vi "Actuators Messenger Template.vi"(0 "Notifier Name":string, 11 "Error In":errorcluster) -> (4 "Notifier Name Out":string, 15 "Error Out":errorcluster)   [LabVIEW 2020]
uses:
  Actuators Controls/Actuators Actions.ctl
  Actuators Controls/Actuators Note Type.ctl
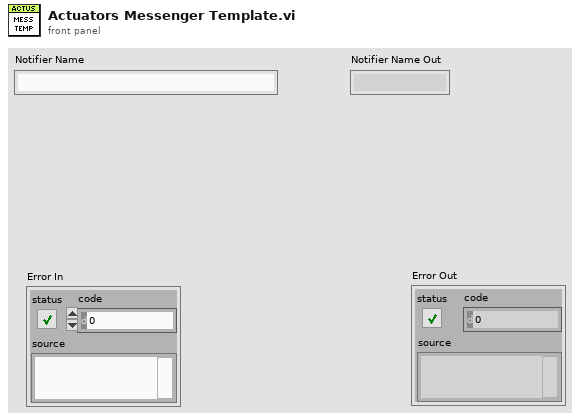
[diagram p1: front panel]
types:
  T1 = typedef "Actuators Note Type.ctl" = cluster{"Actions":T2, "Cmd Received ":bool, "Setpoint":dbl[], "Position":dbl[], "Channel":i32[], "Jog Step":dbl[], "Velocity":dbl[], "Acceleration":dbl[]}
  T2 = typedef "Actuators Actions.ctl" = enum16{"Nothing", "Get Position", "Get Acceleration", "Get Velocity", "Get Jog Step", "Set Acceleration", "Set Velocity", "Set Jog Step", "Move Absolute", "Move Relative", "Jog Forward", "Jog Reverse", "Halt", "Quit"}
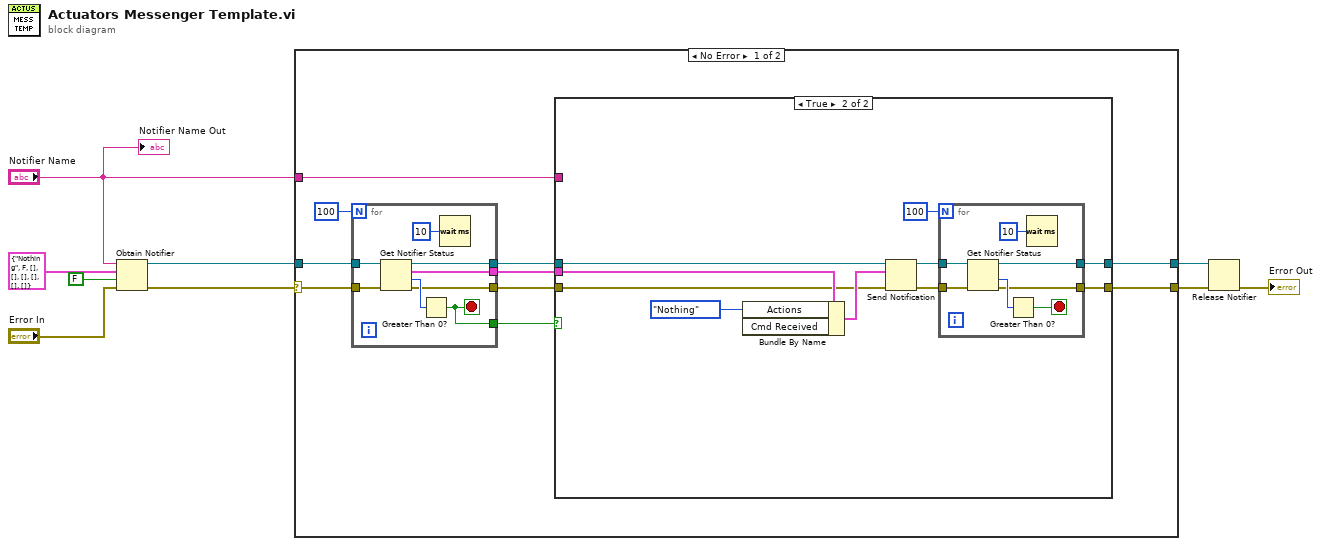
[diagram p0: block diagram]
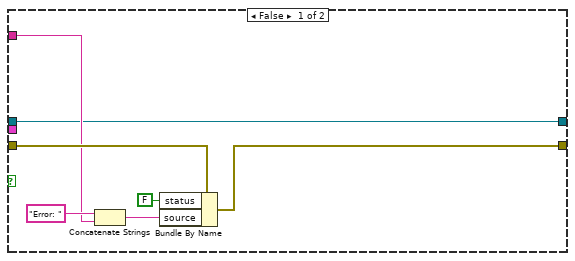
[diagram p2: hidden frame]
diagram:
  n1 = Obtain Notifier(name (unnamed)="Notifier Name", notification data type=T1 {"Actions"=enum."Nothing", "Cmd Received "=FALSE, "Setpoint"=[], "Position"=[], "Channel"=[], "Jog Step"=[], "Velocity"=[], "Acceleration"=[]} ("Actuators Note"), create if not found? (T)=FALSE, error in (no error)="Error In") -> (notifier out=w5:refnum<notifier>, error out=w8:errorcluster)  [unwired: 1 out]
  n2 = case shown="No Error" w8 {
    selector: w8 -> [w17 w52]
    tunnel: w5 -> [w18 w53]
    tunnel: "Notifier Name" -> [w12 _]
    tunnel: [w11 w53] -> w4
    tunnel: [w10 w52] -> w3
    frame No Error {
      n3 = for {
        N: 100 -> [_]
        tunnel: [w50] -> w14
        tunnel: w18 -> [w51]
        tunnel: [w49] -> w15
        tunnel: w17 -> [w46]
        tunnel: [w45] -> w16
        tunnel: [w44] -> w13
        stop <- w45 stop-if-true
        n4 = Get Notifier Status(notifier=w51, error in (no error)=w46) -> (notifier out=w49:refnum<notifier>, current notification=w50:T1, # waiting=w48:i32, error out=w44:errorcluster)  [unwired: 1 out]
        n5 = Greater Than 0?(x=w48) -> (x > 0?=w45:bool)
        n6 = Wait (ms)(milliseconds to wait=u32 10) -> ()  [unwired: 1 out]
      }
      n7 = case shown="True" w16 {
        tunnel: w15 -> [w21 w36]
        tunnel: w14 -> [_ w35]
        tunnel: w13 -> [w26 w32]
        tunnel: w12 -> [w22 _]
        tunnel: [w21 w27] -> w11
        tunnel: [w20 w28] -> w10
        frame False {
          n8 = Concatenate Strings("Error: " ("source"), w22) -> (w23:string)
          n9 = Bundle By Name(cluster=w26, "status"=FALSE, "source"=w23) -> (w20:errorcluster)
        }
        frame True {
          n10 = Bundle By Name(cluster=w35, "Actions"=Actuators_Actions."Nothing") -> (w33:T1)  [unwired: 1 in]
          n11 = Send Notification(notification=w33, notifier=w36, error in (no error)=w32) -> (notifier out=w30:refnum<notifier>, error out=w29:errorcluster)
          n12 = for {
            N: 100 -> [_]
            tunnel: w30 -> [w43]
            tunnel: [w42] -> w27
            tunnel: w29 -> [w39]
            tunnel: [w37] -> w28
            stop <- w38 stop-if-true
            n13 = Get Notifier Status(notifier=w43, error in (no error)=w39) -> (notifier out=w42:refnum<notifier>, # waiting=w41:i32, error out=w37:errorcluster)  [unwired: 2 out]
            n14 = Greater Than 0?(x=w41) -> (x > 0?=w38:bool)
            n15 = Wait (ms)(milliseconds to wait=u32 10) -> ()  [unwired: 1 out]
          }
        }
      }
    }
    frame Error {
    }
  }
  n16 = Release Notifier(notifier=w4, error in (no error)=w3) -> (error out=→"Error Out":errorcluster)  [unwired: 1 in, 2 out]
  "Notifier Name Out" <- "Notifier Name"
